vi "Test 7 compare Diagonally Adjacent symbol.vi"(8 "error in (no error)":errorcluster, 11 "Test Case In":refnum<class "Schema parsing test.lvclass">) -> (0 "error out":errorcluster, 3 "Test Case Out":refnum<class "Schema parsing test.lvclass">)   [LabVIEW 2020, in "Schema parsing test.lvclass"]
uses:
  Schema parsing test.lvclass
  Symbol/Symbol.lvclass
  Number/Number.lvclass
  Schema Parser/Schema Parser.lvclass
  <vilib>/Astemes/LUnit/Test Case.lvclass
  C:/Program Files (x86)/National Instruments/LabVIEW 2020/vi.lib/Astemes/LUnit/Test Case.lvclass
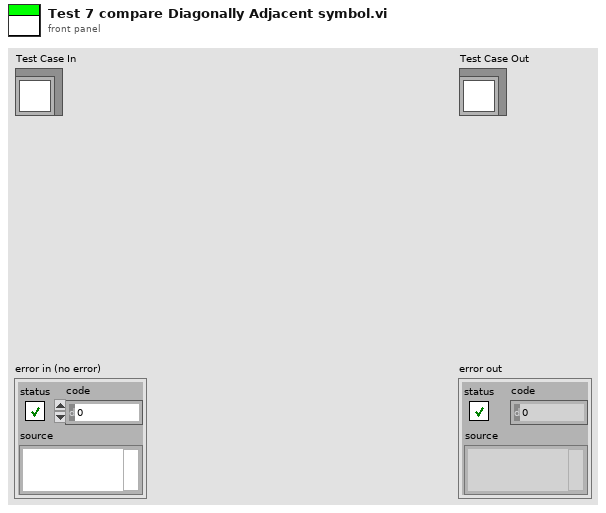
[diagram p1: front panel]
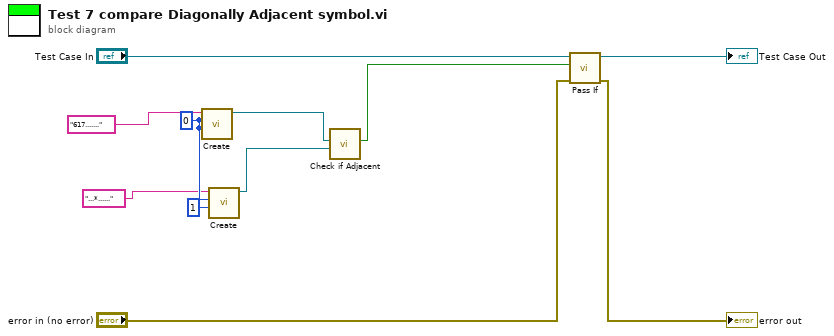
[diagram p0: block diagram]
diagram:
  w6 = 0 ("Col Offset")
  n1 = call "Create.vi"("Row"=w6, "Col Offset"=w6, "String"="617.......") -> ("Number"=w5:refnum<class "Number.lvclass">)  [unwired: 6 in, 2 out]
  n2 = call "Create.vi"("Row"=1, "Col Offset"=w6, "String"="...*......") -> ("Number"=w4:refnum<class "Symbol.lvclass">)  [unwired: 6 in, 2 out]
  n3 = call "Check if Adjacent.vi"("Symbol.lvclass"=w4, "Number.lvclass"=w5) -> ("Is Adjacent?"=w3:bool)  [unwired: 8 in, 1 out]
  n4 = call <vilib>:"Pass If.vi"("error in (no error)"="error in (no error)", "Pass?"=w3, "LUnit Test Case In"="Test Case In") -> ("error out"=→"error out":errorcluster, "LUnit Test Case Out"=→"Test Case Out":refnum<class "Schema parsing test.lvclass">)  [unwired: 7 in]
